vi "Echo Server Main.vi"() -> ()   [LabVIEW 2019]
doc: "<b>Description</b> WebSocket Echo Server example.\n\nBSD 3-Clause License\n\nCopyright (c) 2021, tauterra\nAll rights reserved.\n\nRedistribution and use in source and binary forms, with or without\nmodification, are permitted provided that the following conditions are met:\n\n1. Redistributions of source code must retain the above copyright notice, this\n list of conditions and the following disclaimer.\n\n2. Redistributions in binary form must reproduce the above copyright notice,\n this list of conditions and the following disclaimer in the documentation\n and/or other materials provided with the distribution.\n\n3. Neither the name of the copyright holder nor the names of its\n contributors may be used to endorse or promote products derived from\n this software without specific prior written permission.\n\nTHIS SOFTWARE IS PROVIDED BY THE COPYRIGHT HOLDERS AND CONTRIBUTORS \"AS IS\"\nAND ANY EXPRESS OR IMPLIED WARRANTIES, INCLUDING, BUT NOT LIMITED TO, THE\nIMPLIED WARRANTIES OF MERCHANTABILITY AND FITNESS FOR A PARTICULAR PURPOSE ARE\nDISCLAIMED. IN NO EVENT SHALL THE COPYRIGHT HOLDER OR CONTRIBUTORS BE LIABLE\nFOR ANY DIRECT, INDIRECT, INCIDENTAL, SPECIAL, EXEMPLARY, OR CONSEQUENTIAL\nDAMAGES (INCLUDING, BUT NOT LIMITED TO, PROCUREMENT OF SUBSTITUTE GOODS OR\nSERVICES; LOSS OF USE, DATA, OR PROFITS; OR BUSINESS INTERRUPTION) HOWEVER\nCAUSED AND ON ANY THEORY OF LIABILITY, WHETHER IN CONTRACT, STRICT LIABILITY,\nOR TORT (INCLUDING NEGLIGENCE OR OTHERWISE) ARISING IN ANY WAY OUT OF THE USE\nOF THIS SOFTWARE, EVEN IF ADVISED OF THE POSSIBILITY OF SUCH DAMAGE."
uses:
  WebSocket Echo Server.lvclass
  C:/Users/Nicholas Folse/Documents/workspace/github-tauterra.llc/builds/WebSocketServer Toolkit/TauTerra WebSocketServer Toolkit/TauTerra WebSocketServer Toolkit.lvlibp/classes/WebSocket Connection Handler/WebSocket Connection Handler.lvclass
  TauTerra WebSocketServer Toolkit.lvlibp/classes/WebSocket Queue Logger/WebSocket Queue Logger.lvclass
  C:/Users/Nicholas Folse/Documents/workspace/github-tauterra.llc/builds/WebSocketServer Toolkit/TauTerra WebSocketServer Toolkit/TauTerra WebSocketServer Toolkit.lvlibp/classes/WebSocket Logger/WebSocket Logger.lvclass
  builds/WebSocketServer Toolkit/TauTerra WebSocketServer Toolkit/TauTerra WebSocketServer Toolkit.lvlibp
panel:
  in  "help":string="socket = new WebSocket('ws://localhost:8085'); \nsocket.addEventListener('message', function(evt) {console.log(evt.data);});\n\nsocket.send('hello');\n\nsocket.close()" caption="copy-paste the following commands to a web browser console window..."
  in  "max connections":u32=32
  in  "port":u16=8085
  in  "Log":i32(listbox)=-1
  in  "stop":bool
  # "To test:\nReview example at: \nhttps://developer.mozilla.org/en-US/docs/Web/API/WebSocket"
  # "A WebSocket echo server will be active while this VI is running. \n\nClick 'Stop' to terminate the server."
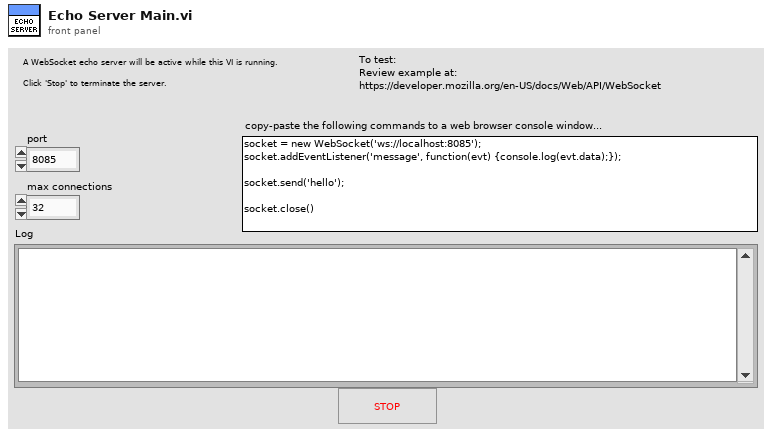
[diagram p1: front panel]
types:
  T1 = enum32{"invalid app kind", "Development System", "Run Time System", "Student Edition", "Embedded LabVIEW", "Evaluation", "Custom"}
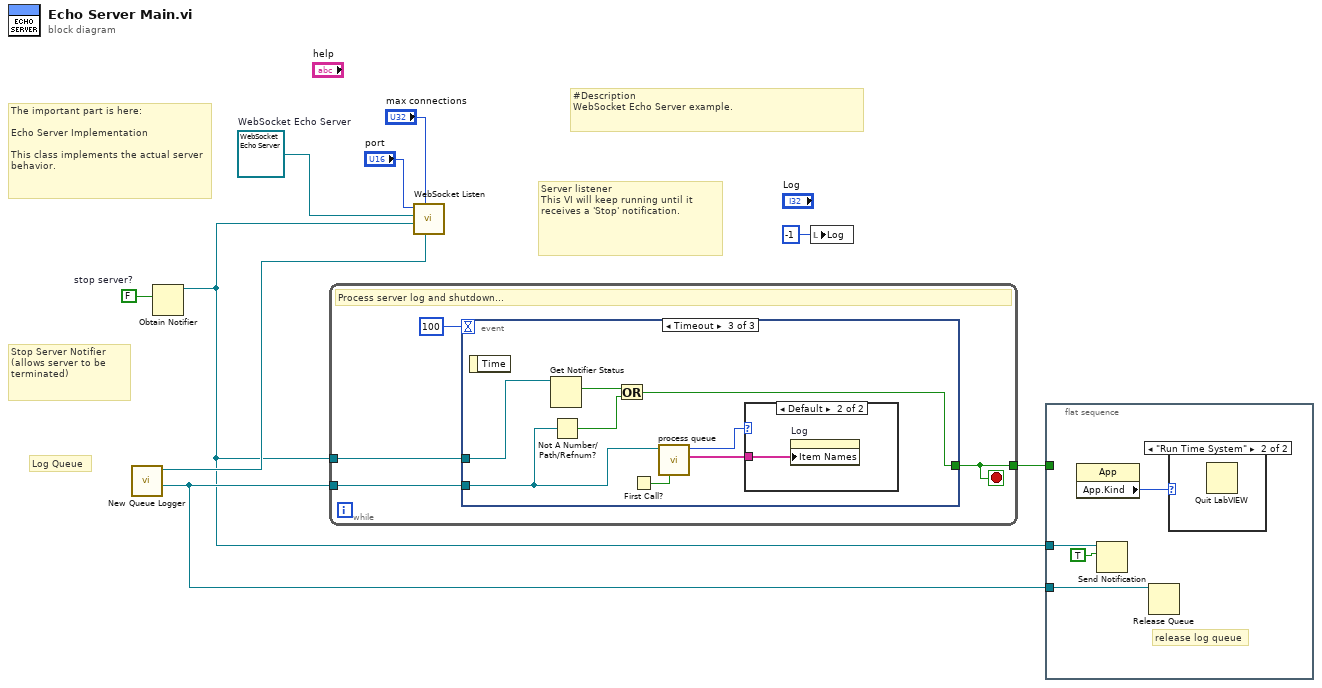
[diagram p0: block diagram]
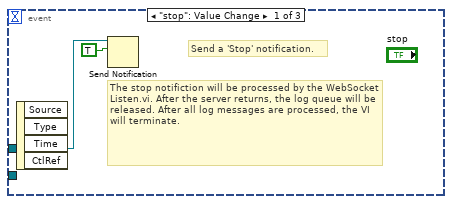
[diagram p3: hidden frame]
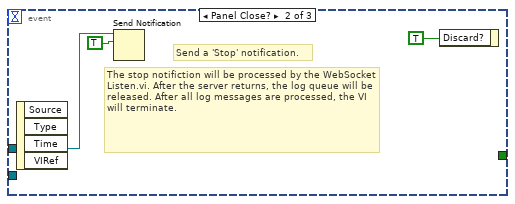
[diagram p4: hidden frame]
diagram:
  w9 = FALSE  # stop server?
  w6 = refnum<class "WebSocket Echo Server.lvclass"> refnum  # WebSocket Echo Server
  # "Server listener\nThis VI will keep running until it receives a 'Stop' notification."
  # "#Description\nWebSocket Echo Server example."
  # "Log Queue"
  # "Stop Server Notifier (allows server to be terminated)"
  # "The important part is here:\n\nEcho Server Implementation\n\nThis class implements the actual server behavior."
  n1 = call "New Queue Logger.vi"() -> ("log queue (out)"=w2:refnum<queue>, "WebSocket Queue Logger out"=w7:refnum<class "WebSocket Queue Logger.lvclass">)  [unwired: 9 in, 1 out]
  n2 = Obtain Notifier(notification data type=w9) -> (notifier out=w1:refnum<notifier>)  [unwired: 3 in, 2 out]
  n3 = while {
    tunnel: w1 -> [w13]
    tunnel: [w12] -> w3
    tunnel: w2 -> [w10]
    stop <- w12 stop-if-true
    # "Process server log and shutdown..."
    n4 = event shown="[2] Timeout" {
      selector: _ -> [_ _ _]
      dyn-events: _ -> [_ _ _]
      timeout: 100 -> [_ _ _]
      tunnel: w13 -> [w15 w18 w23]
      tunnel: [_ _ w22] -> w12
      tunnel: w10 -> [_ _ w26]
      event "stop": Value Change {
        # "The stop notifiction will be processed by the WebSocket Listen.vi. After the server returns, the log queue will be released. After all log messages are processed, the VI will terminate."
        # "Send a 'Stop' notification."
        n5 = event-data() -> ()  [unwired: 1 in, 4 out]
        n6 = Send Notification(notification=TRUE, notifier=w15) -> ()  [unwired: 1 in, 2 out]
      }
      event Panel Close? {
        # "The stop notifiction will be processed by the WebSocket Listen.vi. After the server returns, the log queue will be released. After all log messages are processed, the VI will terminate."
        # "Send a 'Stop' notification."
        n7 = event-data() -> ()  [unwired: 1 in, 4 out]
        n8 = Send Notification(notification=TRUE, notifier=w18) -> ()  [unwired: 1 in, 2 out]
        n9 = event-data("Discard?"=TRUE) -> ()  [unwired: 1 in, 1 out]
      }
      event Timeout {
        n10 = event-data() -> ()  [unwired: 1 in, 1 out]
        n11 = Get Notifier Status(notifier=w23) -> (current notification=w21:bool)  [unwired: 1 in, 4 out]
        n12 = Not A Number/Path/Refnum?(number/path/refnum=w26) -> (NaN/Path/Refnum?=w25:bool)
        n13 = Or(x=w21, y=w25) -> (x .or. y?=w22:bool)
        n14 = First Call?() -> (First Call?: T/F=w19:bool)
        n15 = call "process queue.vi"("clear log?"=w19, "log queue"=w26) -> ("log items"=w20:string[], "# of items retrieved"=w24:i32)  [unwired: 8 in]
        n16 = case shown="Default" w24 {
          tunnel: w20 -> [_ w27]
          frame 0 {
          }
          frame Default {
            n17 = property on="Log" class="LstBox (strict)"("Item Names"=w27) -> ()  [unwired: 2 in, 2 out]
          }
        }
      }
    }
  }
  n18 = call "WebSocket Listen.vi"("WebSocket Logger"=w7, "max connections (32)"="max connections", "quit?"=w1, "WebSocket Connection Handler"=w6, "port"="port") -> ()  [unwired: 6 in, 1 out]
  n19 = local write "Log"(-1 ("Log")) -> ()
  n20 = flat-sequence {
    tunnel: w3 -> [_]
    tunnel: w2 -> [w31]
    tunnel: w1 -> [w30]
    frame #0 {
      # "release log queue"
      n21 = property class="App"() -> ("App.Kind"=w28:T1)  [unwired: 2 in, 2 out]
      n22 = Send Notification(notification=TRUE, notifier=w30) -> ()  [unwired: 1 in, 2 out]
      n23 = Release Queue(queue=w31) -> ()  [unwired: 2 in, 3 out]
      n24 = case shown="\"Run Time System\"" w28 {
        frame Default {
        }
        frame "Run Time System" {
          n25 = Quit LabVIEW() -> ()  [unwired: 1 in]
        }
      }
    }
  }
